vi "run.data_source_count.vi"(8 "error in":errorcluster, 11 "Run in":refnum<class "Run.lvclass">) -> (0 "error out":errorcluster, 3 "Run out":refnum<class "Run.lvclass">)   [LabVIEW 2020, in "Run.lvclass"]
doc: "Returns the number of data sources (datasets, videos, or connections) attached to the run."
uses:
  Run.lvclass
  Run.lvclass/Run.ctl
  client.lvlib
panel:
  out "out_count out":u32
  in  "out_count":u32
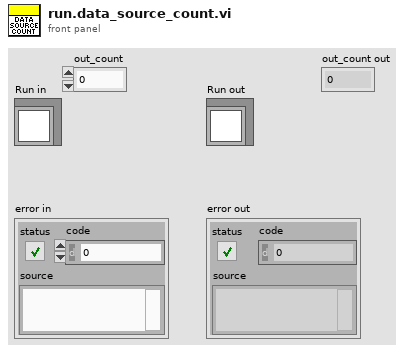
[diagram p1: front panel]
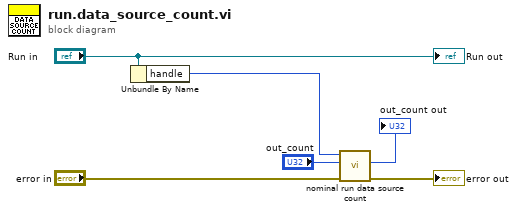
[diagram p0: block diagram]
diagram:
  n1 = Unbundle By Name("Run in") -> ("handle"=w4:i32)
  n2 = call "nominal run data source count.vi"("error in (no error)"="error in", "out_count"="out_count", "run"=w4) -> ("error out"=→"error out":errorcluster, "out_count out"=→"out_count out":u32)  [unwired: 6 in, 1 out]
  "Run out" <- "Run in"
